vi "swap tracking spot.vi"(0 "N spot tracker in":T5, 1 "tracking state in":T6={"x state"={"pos estimate"=0.0, "v estimate"=0.0, "weighted position error sum"=0.0, "photon count"=0, "transmit tick count"=0, "axis number"=0, "px (levels^2)"=0.0, "pxv (levels^2/ticks)"=0.0, "pv (levels^2/ticks^2)"=0.0, "vel diff (levels^2/ticks^3)"=0.0, "gx"=0.0, "rtwiddle"=0.0, "photon count ch0"=0, "photon count ch1"=0, "Dx -levels^2/ticks"=0.0}, "y state"={"pos estimate"=0.0, "v estimate"=0.0, "weighted position error sum"=0.0, "photon count"=0, "transmit tick count"=0, "axis number"=1, "px (levels^2)"=0.0, "pxv (levels^2/ticks)"=0.0, "pv (levels^2/ticks^2)"=0.0, "vel diff (levels^2/ticks^3)"=0.0, "gx"=0.0, "rtwiddle"=0.0, "photon count ch0"=0, "photon count ch1"=0, "Dx -levels^2/ticks"=0.0}, "z state"={"pos estimate"=0.0, "v estimate"=0.0, "weighted position error sum"=0.0, "photon count"=0, "transmit tick count"=0, "axis number"=2, "px (levels^2)"=0.0, "pxv (levels^2/ticks)"=0.0, "pv (levels^2/ticks^2)"=0.0, "vel diff (levels^2/ticks^3)"=0.0, "gx"=0.0, "rtwiddle"=0.0, "photon count ch0"=0, "photon count ch1"=0, "Dx -levels^2/ticks"=0.0}, "spot number"=0}, 2 "bleach mode":bool, 3 "reset flags":u8, 4 "new circle":bool, 5 "permission to swap states":bool, 6 "tracking?":bool=TRUE, 7 "spot location constraints":T3=[{"spot number"=0, "active"=FALSE, "x max"=0, "x min"=0, "y max"=0, "y min"=0}, {"spot number"=0, "active"=FALSE, "x max"=0, "x min"=0, "y max"=0, "y min"=0}, {"spot number"=0, "active"=FALSE, "x max"=0, "x min"=0, "y max"=0, "y min"=0}, {"spot number"=0, "active"=FALSE, "x max"=0, "x min"=0, "y max"=0, "y min"=0}], 8 "pockels normal":i16, 9 "pockels bleach":i16, 10 "current location":T2, 11 "update tracking? in":T1, 12 "pockels always on":bool, 13 "ff vel?":bool) -> (14 "N spot tracker out":T5, 15 "tracking state out":T6={"x state"={"pos estimate"=0.0, "v estimate"=0.0, "weighted position error sum"=0.0, "photon count"=0, "transmit tick count"=0, "axis number"=0, "px (levels^2)"=0.0, "pxv (levels^2/ticks)"=0.0, "pv (levels^2/ticks^2)"=0.0, "vel diff (levels^2/ticks^3)"=0.0, "gx"=0.0, "rtwiddle"=0.0, "photon count ch0"=0, "photon count ch1"=0, "Dx -levels^2/ticks"=0.0}, "y state"={"pos estimate"=0.0, "v estimate"=0.0, "weighted position error sum"=0.0, "photon count"=0, "transmit tick count"=0, "axis number"=1, "px (levels^2)"=0.0, "pxv (levels^2/ticks)"=0.0, "pv (levels^2/ticks^2)"=0.0, "vel diff (levels^2/ticks^3)"=0.0, "gx"=0.0, "rtwiddle"=0.0, "photon count ch0"=0, "photon count ch1"=0, "Dx -levels^2/ticks"=0.0}, "z state"={"pos estimate"=0.0, "v estimate"=0.0, "weighted position error sum"=0.0, "photon count"=0, "transmit tick count"=0, "axis number"=2, "px (levels^2)"=0.0, "pxv (levels^2/ticks)"=0.0, "pv (levels^2/ticks^2)"=0.0, "vel diff (levels^2/ticks^3)"=0.0, "gx"=0.0, "rtwiddle"=0.0, "photon count ch0"=0, "photon count ch1"=0, "Dx -levels^2/ticks"=0.0}, "spot number"=0}, 16 "update tracking? out":T1, 17 "pockels voltage":i16, 18 "use photons to track":bool)   [LabVIEW 2010]
uses:
  kalman 3-axis state.ctl
  integrating single axis kalman state.ctl
  kalman N spot state.ctl
  spot location constraints.ctl
  spot location constraint.ctl
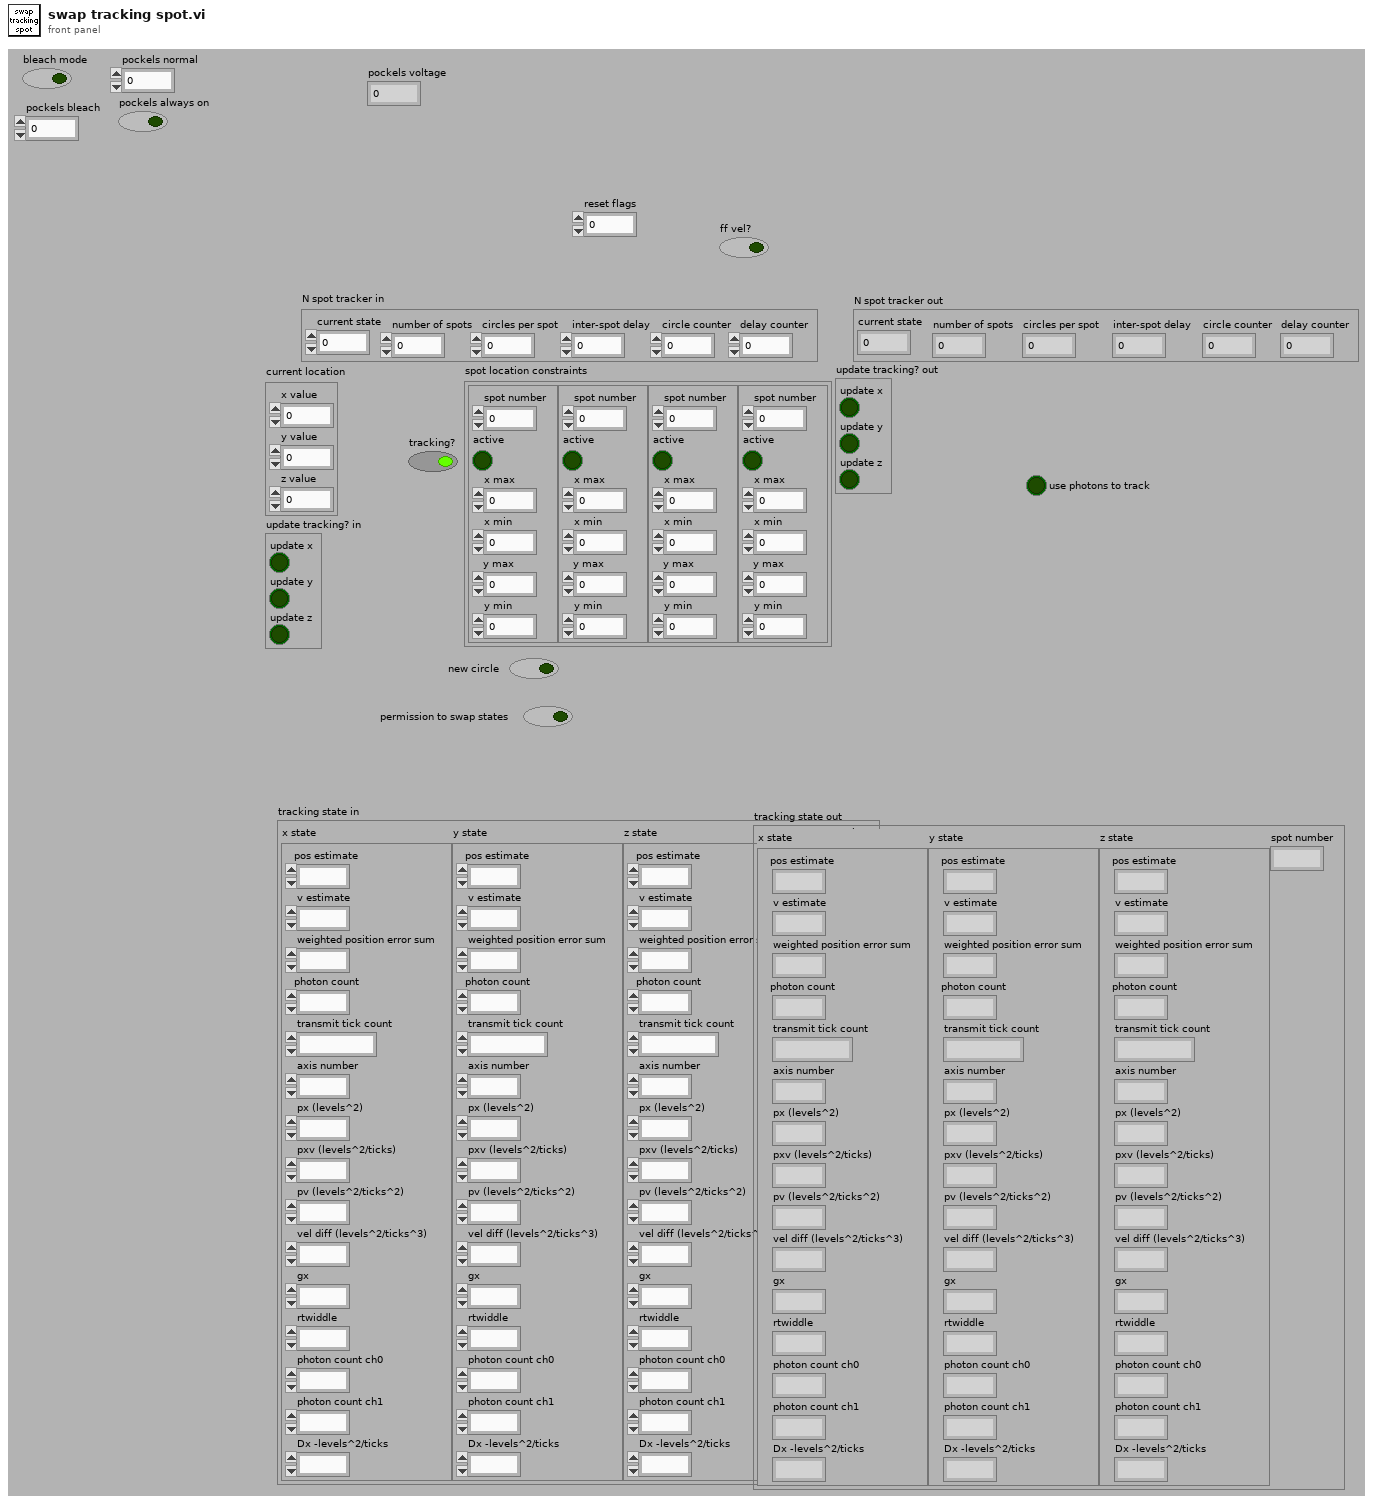
[diagram p1: front panel]
types:
  T1 = cluster{"update x":bool, "update y":bool, "update z":bool}
  T2 = cluster{"x value":i16, "y value":i16, "z value":i16}
  T3 = typedef "spot location constraints.ctl" = T4[]
  T4 = typedef "spot location constraint.ctl" = cluster{"spot number":i8, "active":bool, "x max":i16, "x min":i16, "y max":i16, "y min":i16}
  T5 = typedef "kalman N spot state.ctl" = cluster{"current state":u8, "number of spots":u8, "circles per spot":u16, "inter-spot delay":u8, "circle counter":u16, "delay counter":u8}
  T6 = typedef "kalman 3-axis state.ctl" = cluster{"x state":T7, "y state":T7, "z state":T7, "spot number":u8}
  T7 = typedef "integrating single axis kalman state.ctl" = cluster{"pos estimate":fxp<+/-,32,16>, "v estimate":fxp<+/-,16,0>, "weighted position error sum":fxp<+/-,32,32>, "photon count":u32, "transmit tick count":u32, "axis number":u8, "px (levels^2)":fxp<+,32,19>, "pxv (levels^2/ticks)":fxp<+,32,2>, "pv (levels^2/ticks^2)":fxp<+,32,-14>, "vel diff (levels^2/ticks^3)":fxp<+,24,-22>, "gx":fxp<+,16,8>, "rtwiddle":fxp<+,16,26>, "photon count ch0":u32, "photon count ch1":u32, "Dx -levels^2/ticks":fxp<+,32,19>}
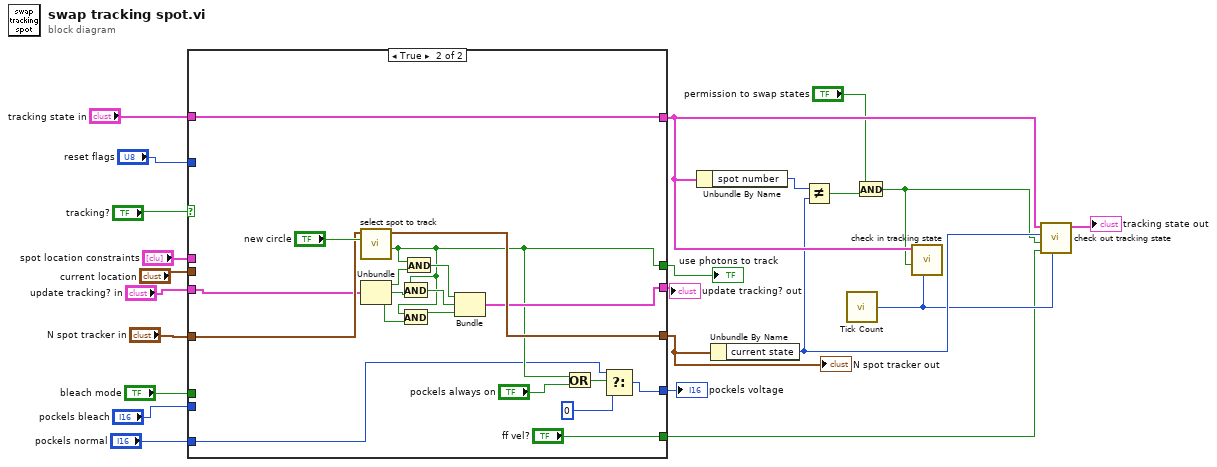
[diagram p0: block diagram]
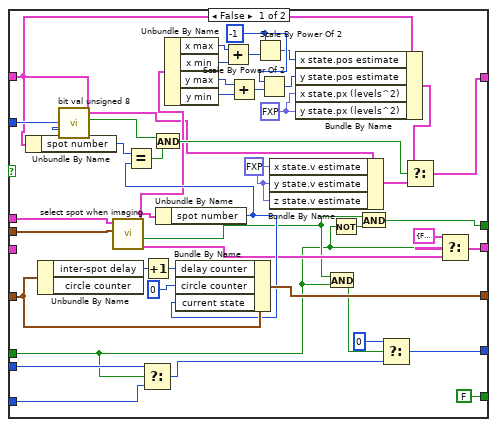
[diagram p2: hidden frame]
diagram:
  n1 = case shown="True" "tracking?" {
    tunnel: [w30 w73] -> w21
    tunnel: [w62 w84] -> w20
    tunnel: "N spot tracker in" -> [w63 w83]
    tunnel: "spot location constraints" -> [w61 _]
    tunnel: "current location" -> [w60 _]
    tunnel: [w38 w74] -> w17
    tunnel: "update tracking? in" -> [_ w81]
    tunnel: "tracking state in" -> [w42 w82]
    tunnel: [w40 w82] -> w12
    tunnel: "reset flags" -> [w55 _]
    tunnel: "bleach mode" -> [w28 _]
    tunnel: "pockels bleach" -> [w36 _]
    tunnel: "pockels normal" -> [w35 w70]
    tunnel: [w31 w68] -> w2
    tunnel: [FALSE ("ff vel?") "ff vel?"] -> w1
    frame False {
      w25 = fxp<+/-,16,0> 0.0 ("x state.v estimate")
      w41 = fxp<+,32,19> 0.0 ("x state.px (levels^2)")
      w46 = -1 ("n")
      n2 = Unbundle By Name(w42) -> ("spot number"=w56:u8)
      n3 = Unbundle By Name(w63) -> ("inter-spot delay"=w66:u8)  [unwired: 1 out]
      n4 = call "bit val unsigned 8.vi"("bit num"=w56, "x"=w55) -> ("BV"=w57:bool)  [unwired: 9 in]
      n5 = call "select spot when imaging.vi"("current location"=w60, "spot location constraints"=w61) -> ("update tracking?"=w39:T1, "use photons to track"=w29:bool, "selected spot"=w53:T4)  [unwired: 7 in]
      n6 = Select(t=w36, s=w28, f=w35) -> (s? t:f=w33:i16)
      n7 = Increment(x=w66) -> (x+1=w65:u8)
      n8 = Unbundle By Name(w53) -> ("spot number"=w59:i8)
      n9 = Equal?(x=w56, y=w59) -> (x = y?=w58:bool)
      n10 = And(x=w57, y=w58) -> (x .and. y?=w54:bool)
      n11 = Unbundle By Name(w53) -> ("x max"=w51:i16, "x min"=w52:i16, "y max"=w50:i16, "y min"=w49:i16)
      n12 = Bundle By Name(cluster=w63, "delay counter"=w65, "circle counter"=u8 0, "current state"=w59) -> (w62:T5)
      n13 = Add(x=w51, y=w52) -> (x+y=w48:i16)
      n14 = Add(x=w50, y=w49) -> (x+y=w47:i16)
      n15 = Scale By Power Of 2(n=w46, x=w48) -> (x*2^n=w45:i16)
      n16 = Scale By Power Of 2(n=w46, x=w47) -> (x*2^n=w44:i16)
      n17 = Bundle By Name(cluster=w42, "x state.v estimate"=w25, "y state.v estimate"=w25, "z state.v estimate"=w25) -> (w26:T6)
      n18 = Bundle By Name(cluster=w42, "x state.pos estimate"=w45, "y state.pos estimate"=w44, "x state.px (levels^2)"=w41, "y state.px (levels^2)"=w41) -> (w43:T6)
      n19 = And(x=w29, y=w28) -> (x .and. y?=w34:bool)
      n20 = Not(x=w28) -> (.not. x?=w27:bool)
      n21 = And(x=w29, y=w27) -> (x .and. y?=w30:bool)
      n22 = Select(t=i16 0, s=w34, f=w33) -> (s? t:f=w31:i16)
      n23 = Select(t=w43, s=w54, f=w26) -> (s? t:f=w40:T6)
      n24 = Select(t=T1 {"update x"=FALSE, "update y"=FALSE, "update z"=FALSE}, s=w28, f=w39) -> (s? t:f=w38:T1)
    }
    frame True {
      n25 = call "select spot to track.vi"("new circle"="new circle", "N spot tracker in"=w83) -> ("use photons to track"=w73:bool, "N spot tracker out"=w84:T5)  [unwired: 8 in]
      n26 = Unbundle(w81) -> ("update x"=w80:bool, "update y"=w79:bool, "update z"=w78:bool)
      n27 = And(x=w73, y=w79) -> (x .and. y?=w76:bool)
      n28 = And(x=w73, y=w78) -> (x .and. y?=w75:bool)
      n29 = And(x=w73, y=w80) -> (x .and. y?=w77:bool)
      n30 = Bundle(w77, w76, w75) -> (w74:cluster{bool, bool, bool})  [unwired: 1 in]
      n31 = Or(x=w73, y="pockels always on") -> (x .or. y?=w72:bool)
      n32 = Select(t=w70, s=w72, f=i16 0) -> (s? t:f=w68:i16)
    }
  }
  "use photons to track" <- w21
  "N spot tracker out" <- w20
  "update tracking? out" <- w17
  "pockels voltage" <- w2
  n33 = Unbundle By Name(w12) -> ("spot number"=w11:u8)
  n34 = Unbundle By Name(w20) -> ("current state"=w10:u8)
  n35 = Not Equal?(x=w11, y=w10) -> (x != y?=w9:bool)
  n36 = call "Tick Count"() -> ("Tick Count(Ticks)"=w6:u32)
  n37 = And(x="permission to swap states", y=w9) -> (x .and. y?=w7:bool)
  n38 = call "check in tracking state.vi"("tick count"=w6, "check in state"=w7, "state to check in"=w12) -> ()  [unwired: 9 in]
  n39 = call "check out tracking state.vi"("tick count"=w6, "ff vel?"=w1, "check out state"=w7, "state number"=w10, "previous state"=w12) -> ("state out"=→"tracking state out":T6)  [unwired: 6 in]
